vi "Webservice for-LV-and-python-template.vi"() -> ()   [LabVIEW 2018]
uses:
  <vilib>/Utility/error.llb/DialogType.ctl
  <vilib>/httpClient/POSTBuffer.vi
  <vilib>/httpClient/LabVIEWHTTPClient.lvlib
panel:
  in  "String":string="RickyS"
  in  "Numeric":i32=20
  out "standard output":string
  out "standard error":string
  out "body 3":string
  out "GET_ function":string
  out "POST_ function":string
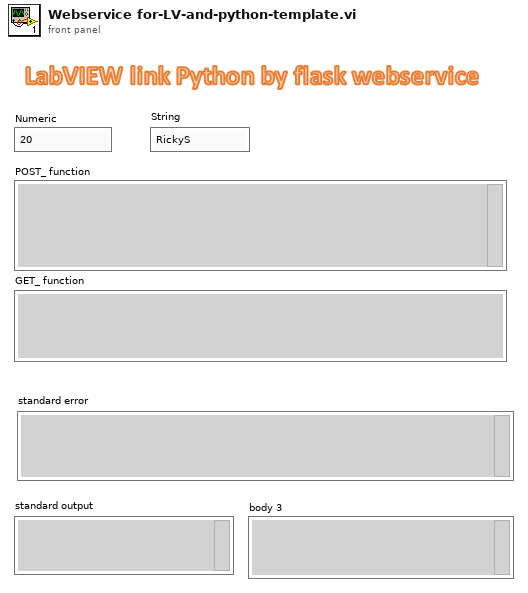
[diagram p1: front panel]
types:
  T1 = typedef "DialogType.ctl" = u16
  T2 = typedef "LabVIEWHTTPClient.lvlib/ClientHandle.ctl" = refnum<k1>
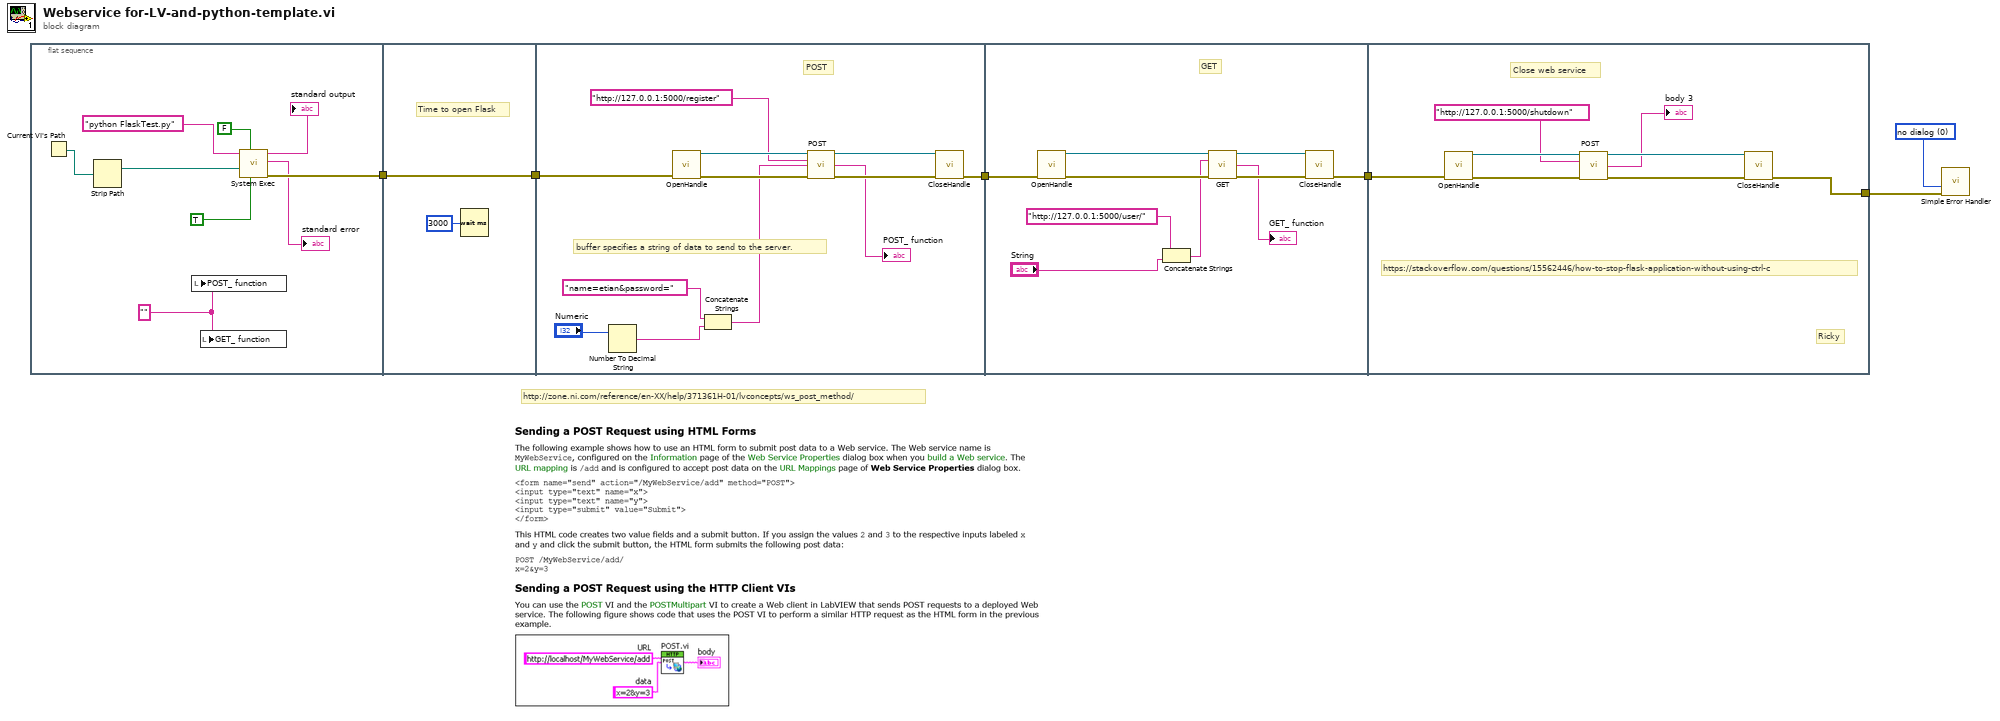
[diagram p0: block diagram]
diagram:
  w3 = T1 0 items=["no dialog", "OK message", "continue or stop message", "OK message + warnings", "continue/stop + warnings"] ("type of dialog (OK msg:1)")
  # "http://zone.ni.com/reference/en-XX/help/371361H-01/lvconcepts/ws_post_method/"
  n1 = flat-sequence {
    tunnel: [w15] -> w2
    tunnel: w2 -> [w17]
    tunnel: [w17] -> w1
    tunnel: [w23] -> w6
    tunnel: w1 -> [w22]
    tunnel: w6 -> [w39]
    tunnel: [w33] -> w5
    tunnel: w5 -> [w41]
    tunnel: [w40] -> w4
    frame #0 {
      w7 = "" ("body")
      n2 = Current VI's Path() -> (path=w14:path)
      n3 = Strip Path(path=w14) -> (stripped path=w13:path)  [unwired: 1 out]
      n4 = local write "POST_ function"(w7) -> ()
      n5 = local write "GET_ function"(w7) -> ()
      n6 = call <vilib>:"System Exec.vi"("run minimized? (F)"=TRUE, "wait until completion? (T)"=FALSE, "working directory"=w13, "command line"="python FlaskTest.py") -> ("error out"=w15:errorcluster, "standard error"=→"standard error":string, "standard output"=→"standard output":string)  [unwired: 4 in, 1 out]
    }
    frame #1 {
      # "Time to open Flask"
      n7 = Wait (ms)(milliseconds to wait=u32 3000) -> ()  [unwired: 1 out]
    }
    frame #2 {
      # "POST"
      # "buffer specifies a string of data to send to the server."
      n8 = Number To Decimal String(number="Numeric") -> (decimal integer string=w19:string)  [unwired: 1 in]
      n9 = call <vilib>:"OpenHandle.vi"("error in (no error)"=w22) -> ("client handle out"=w29:T2, "error out"=w27:errorcluster)  [unwired: 13 in]
      n10 = Concatenate Strings("name=etian&password=" ("buffer"), w19) -> (w18:string)
      n11 = call-poly <vilib>:"POST.vi"("client handle"=w29, "url"="http://127.0.0.1:5000/register", "buffer"=w18, "error in (no error)"=w27) -> ("client handle out"=w28:T2, "body"=→"POST_ function":string, "error out"=w26:errorcluster)  [unwired: 8 in, 1 out]
      n12 = call <vilib>:"CloseHandle.vi"("client handle"=w28, "error in (no error)"=w26) -> ("error out"=w23:errorcluster)  [unwired: 13 in]
    }
    frame #3 {
      # "GET"
      n13 = call <vilib>:"OpenHandle.vi"("error in (no error)"=w39) -> ("client handle out"=w35:T2, "error out"=w38:errorcluster)  [unwired: 13 in]
      n14 = Concatenate Strings("http://127.0.0.1:5000/user/" ("url"), "String") -> (w30:string)
      n15 = call <vilib>:"GET.vi"("client handle"=w35, "url"=w30, "error in (no error)"=w38) -> ("client handle out"=w34:T2, "body"=→"GET_ function":string, "error out"=w37:errorcluster)  [unwired: 9 in, 1 out]
      n16 = call <vilib>:"CloseHandle.vi"("client handle"=w34, "error in (no error)"=w37) -> ("error out"=w33:errorcluster)  [unwired: 13 in]
    }
    frame #4 {
      # "Close web service"
      # "Ricky"
      # "https://stackoverflow.com/questions/15562446/how-to-stop-flask-application-without-using-ctrl-c"
      n17 = call <vilib>:"OpenHandle.vi"("error in (no error)"=w41) -> ("client handle out"=w47:T2, "error out"=w45:errorcluster)  [unwired: 13 in]
      n18 = call-poly <vilib>:"POST.vi"("client handle"=w47, "url"="http://127.0.0.1:5000/shutdown", "error in (no error)"=w45) -> ("client handle out"=w46:T2, "body"=→"body 3":string, "error out"=w44:errorcluster)  [unwired: 9 in, 1 out]
      n19 = call <vilib>:"CloseHandle.vi"("client handle"=w46, "error in (no error)"=w44) -> ("error out"=w40:errorcluster)  [unwired: 13 in]
    }
  }
  n20 = call <vilib>:"Simple Error Handler.vi"("type of dialog (OK msg:1)"=w3, "error in (no error)"=w4) -> ()  [unwired: 3 in, 5 out]
